vi "IT.vi"(7 "error in (no error)":errorcluster, 10 "機號":string) -> (0 "error out":errorcluster, 1 "Msg":string, 2 "BARCODE":string, 3 "Date Time":string, 4 "UP OK":bool)   [LabVIEW 2014]
uses:
  C:/Program Files (x86)/National Instruments/LabVIEW 2014/user.lib/WebService/_WMIM9900/WMIM9900.dll
  Program Files (x86)/National Instruments/LabVIEW 2014/user.lib/WebService/_WMIM9900/WMIM9900.dll
panel:
  in  "Proxy Server Settings":T1={"Address"="10.90.118.10", "Port"=80, "Username"="", "Password"="", "Domain"=""}
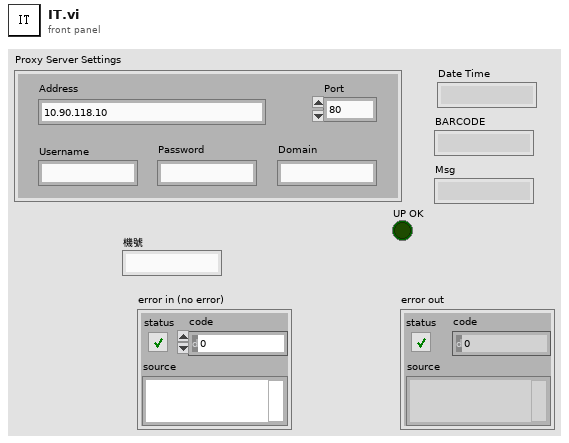
[diagram p1: front panel]
types:
  T1 = cluster{"Address":string, "Port":u32, "Username":string, "Password":string, "Domain":string}
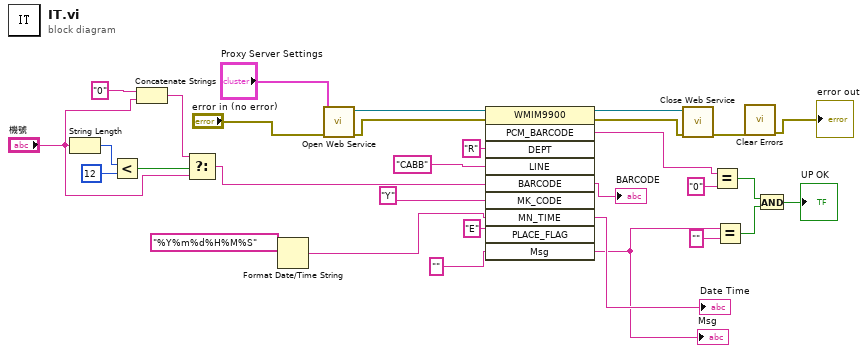
[diagram p0: block diagram]
diagram:
  n1 = String Length(string="機號") -> (length=w7:i32)
  n2 = Less?(x=w7, y=12) -> (x < y?=w5:bool)
  n3 = Concatenate Strings("0" ("string"), "機號") -> (w4:string)
  n4 = Select(t=w4, s=w5, f="機號") -> (s? t:f=w1:string)
  n5 = Format Date/Time String(time format string (%c)="%Y%m%d%H%M%S") -> (date/time string=w25:string)  [unwired: 2 in]
  n6 = call <userlib>:"Open Web Service.vi"("error in (no error)"="error in (no error)", "Proxy Server Settings"="Proxy Server Settings") -> ("error out"=w18:errorcluster, "WMIM9900 refnum"=w31:refnum<k24>)  [unwired: 8 in]
  n7 = invoke class="WMIM9900" method="PCM_BARCODE"(reference=w31, error in=w18, "DEPT"="R", "LINE"="CABB", "BARCODE"=w1, "MK_CODE"="Y", "MN_TIME"=w25, "PLACE_FLAG"="E", "Msg"="") -> (reference out=w30:refnum<k24>, error out=w17:errorcluster, "PCM_BARCODE"=w23:string, "BARCODE"=→"BARCODE":string, "MN_TIME"=→"Date Time":string, "Msg"=w9:string)  [unwired: 1 in, 4 out]
  "Msg" <- w9
  n8 = call <userlib>:"Close Web Service.vi"("error in (no error)"=w17, "WMIM9900 refnum"=w30) -> ("error out"=w13:errorcluster)  [unwired: 9 in]
  n9 = Equal?(x=w23, y="0") -> (x = y?=w21:bool)
  n10 = Equal?(x=w9, y="") -> (x = y?=w20:bool)
  n11 = call <vilib>:"Clear Errors.vi"("error in (no error)"=w13) -> ("error out"=→"error out":errorcluster)  [unwired: 5 in, 1 out]
  n12 = And(x=w21, y=w20) -> (x .and. y?=→"UP OK":bool)
